vi "Running GCODE.vi"(6 "Message Data":variant, 7 "G-Code Array in":string[](array[string]), 8 "error in (no error)":errorcluster, 9 "Cluster in":T1, 10 "dup Message Queue":refnum<queue>) -> (0 "error out":errorcluster, 1 "G-Code Array out":string[](array[string]), 2 "String":string, 3 "Cluster out":T1)   [LabVIEW 2021]
uses:
  support/Message Queue/Message Cluster.ctl
  support/Message Queue/Enqueue Message (Single).vi
  support/Message Queue/Message Queue.lvlib
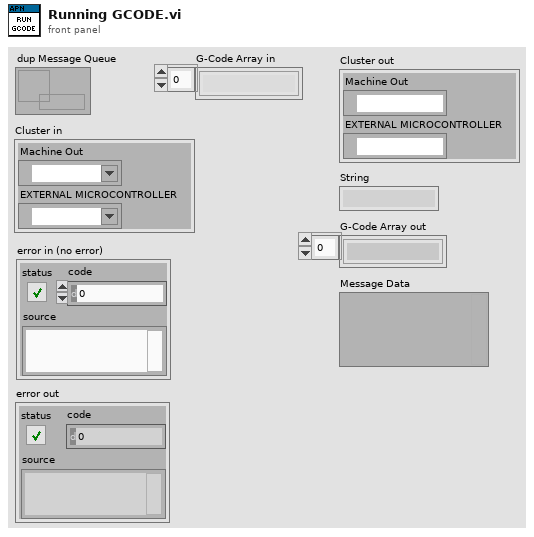
[diagram p1: front panel]
types:
  T1 = cluster{"Machine Out":refnum<visa-resource-name>, "EXTERNAL MICROCONTROLLER":refnum<visa-resource-name>}
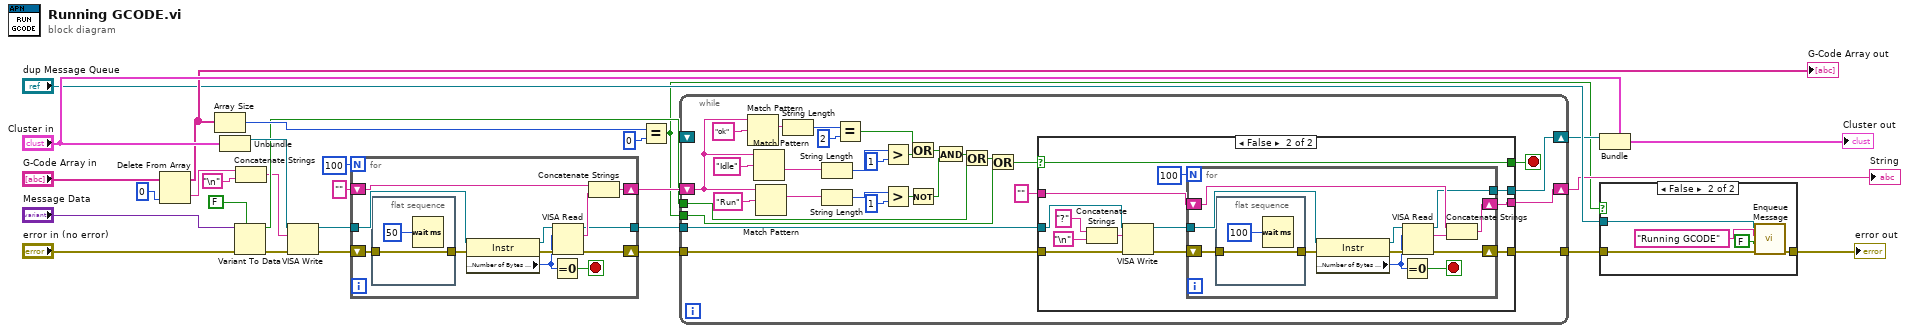
[diagram p0: block diagram]
diagram:
  n1 = Delete From Array(array="G-Code Array in", index=0) -> (deleted portion=w7:string, array with subset deleted=w16:string[])  [unwired: 1 in]
  "G-Code Array out" <- w16
  n2 = Array Size(array=w16) -> (size(s)=w17:i32)
  n3 = Unbundle("Cluster in") -> ("Machine Out"=w23:refnum<visa-resource-name>)  [unwired: 1 out]
  n4 = Variant To Data(error in="error in (no error)", type=FALSE, Variant="Message Data") -> (data=w12:bool, error out=w24:errorcluster)
  n5 = Concatenate Strings(w7, "\n") -> (w6:string)
  n6 = VISA Write(VISA resource name=w23, write buffer=w6, error in (no error)=w24) -> (VISA resource name out=w27:refnum<visa-resource-name>, error out=w28:errorcluster)  [unwired: 1 out]
  n7 = for {
    N: 100 -> [_]
    tunnel: w27 -> [w38]
    shift-right: [w41] -> w29
    shift-left: "" -> [w40]
    shift-right: [w35] -> w2
    shift-left: w28 -> [w33]
    tunnel: [w30] -> w5
    stop <- w31 stop-if-true
    n8 = flat-sequence {
      tunnel: w33 -> [w42]
      tunnel: [w42] -> w32
      frame #0 {
        n9 = Wait (ms)(milliseconds to wait=u32 50) -> ()  [unwired: 1 out]
      }
    }
    n10 = property class="Instr"(reference=w38, error in=w32) -> (reference out=w34:refnum<visa-resource-name>, error out=w39:errorcluster, "Serial Settings:Number of Bytes at Serial Port"=w36:u32)
    n11 = Equal To 0?(x=w36) -> (x = 0?=w31:bool)
    n12 = VISA Read(VISA resource name=w34, byte count=w36, error in (no error)=w39) -> (VISA resource name out=w30:refnum<visa-resource-name>, read buffer=w37:string, error out=w35:errorcluster)  [unwired: 1 out]
    n13 = Concatenate Strings(w40, w37) -> (w41:string)
  }
  n14 = Equal?(x=w17, y=0) -> (x = y?=w3:bool)
  n15 = while {
    tunnel: w3 -> [w73]
    tunnel: w12 -> [w71]
    shift-right: [w60] -> w9
    shift-left: w29 -> [w49]
    tunnel: w5 -> [w57]
    shift-right: [w56] -> w4
    shift-left: _ -> [_]
    tunnel: w2 -> [w55]
    tunnel: [w54] -> w1
    stop <- w58 stop-if-true
    n16 = Match Pattern(string=w49, regular expression="ok") -> (match substring=w61:string)  [unwired: 1 in, 3 out]
    n17 = Match Pattern(string=w49, regular expression="Idle") -> (after substring=w65:string)  [unwired: 1 in, 3 out]
    n18 = Match Pattern(string=w49, regular expression="Run") -> (match substring=w51:string)  [unwired: 1 in, 3 out]
    n19 = String Length(string=w61) -> (length=w66:i32)
    n20 = String Length(string=w65) -> (length=w64:i32)
    n21 = String Length(string=w51) -> (length=w50:i32)
    n22 = Equal?(x=w66, y=2) -> (x = y?=w63:bool)
    n23 = Greater?(x=w64, y=1) -> (0:w62:bool)
    n24 = Greater?(x=w50, y=1) -> (0:w45:bool)
    n25 = Or(x=w63, y=w62) -> (x .or. y?=w47:bool)
    n26 = Not(x=w45) -> (.not. x?=w46:bool)
    n27 = And(x=w47, y=w46) -> (x .and. y?=w48:bool)
    n28 = Or(x=w48, y=w71) -> (x .or. y?=w72:bool)
    n29 = Or(x=w72, y=w73) -> (x .or. y?=w59:bool)
    n30 = case shown="False" w59 {
      selector: w59 -> [w76 w82]
      tunnel: "" -> [w77 w84]
      tunnel: [w77 w83] -> w60
      tunnel: [w76 w82] -> w58
      tunnel: w57 -> [w75 w81]
      tunnel: [w75 w80] -> w56
      tunnel: w55 -> [w74 w79]
      tunnel: [w74 w78] -> w54
      frame True {
      }
      frame False {
        n31 = Concatenate Strings("?" ("string"), "\n") -> (w90:string)
        n32 = VISA Write(VISA resource name=w81, write buffer=w90, error in (no error)=w79) -> (VISA resource name out=w89:refnum<visa-resource-name>, error out=w88:errorcluster)  [unwired: 1 out]
        n33 = for {
          N: 100 -> [_]
          tunnel: w89 -> [w99]
          shift-right: [w102] -> w83
          shift-left: w84 -> [w101]
          shift-right: [w96] -> w78
          shift-left: w88 -> [w94]
          tunnel: [w91] -> w80
          stop <- w92 stop-if-true
          n34 = flat-sequence {
            tunnel: w94 -> [w103]
            tunnel: [w103] -> w93
            frame #0 {
              n35 = Wait (ms)(milliseconds to wait=u32 100) -> ()  [unwired: 1 out]
            }
          }
          n36 = property class="Instr"(reference=w99, error in=w93) -> (reference out=w95:refnum<visa-resource-name>, error out=w100:errorcluster, "Serial Settings:Number of Bytes at Serial Port"=w97:u32)
          n37 = Equal To 0?(x=w97) -> (x = 0?=w92:bool)
          n38 = VISA Read(VISA resource name=w95, byte count=w97, error in (no error)=w100) -> (VISA resource name out=w91:refnum<visa-resource-name>, read buffer=w98:string, error out=w96:errorcluster)  [unwired: 1 out]
          n39 = Concatenate Strings(w101, w98) -> (w102:string)
        }
      }
    }
  }
  "String" <- w9
  n40 = Bundle(cluster="Cluster in", "Machine Out"=w4) -> (→"Cluster out":T1)  [unwired: 1 in]
  n41 = case shown="False" w3 {
    tunnel: w1 -> [w105 w110]
    tunnel: [w105 w109] -> w22
    tunnel: "dup Message Queue" -> [_ w108]
    frame True {
    }
    frame False {
      n42 = call-poly "Enqueue Message.vi"("error in (no error)"=w110, "Message Data"=FALSE ("x = y?"), "Message"="Running GCODE", "Message Queue"=w108) -> ("error out"=w109:errorcluster)  [unwired: 6 in, 1 out]
    }
  }
  "error out" <- w22
